vi "Read Constants.vi"(8 "error in (no error)":errorcluster, 11 "Tank Drive in":refnum<class "Tank Drive.lvclass">) -> (0 "error out":errorcluster, 2 "Constants":T1={"Drive Velocity Low Gear"={"P"=0.0, "I"=0.0, "D"=0.0, "F"=0.0, "integralZone"=0.0, "allowableClosedLoopError"=0, "maxIntegralAccumulator"=0.0, "closedLoopPeakOutput"=1.0, "closedLoopPeriod"=1}, "Drive Velocity High Gear"={"P"=0.0, "I"=0.0, "D"=0.0, "F"=0.0, "integralZone"=0.0, "allowableClosedLoopError"=0, "maxIntegralAccumulator"=0.0, "closedLoopPeakOutput"=1.0, "closedLoopPeriod"=1}, "Drive Motion Magic Primary Low Gear"={"P"=0.0, "I"=0.0, "D"=0.0, "F"=0.0, "integralZone"=0.0, "allowableClosedLoopError"=0, "maxIntegralAccumulator"=0.0, "closedLoopPeakOutput"=1.0, "closedLoopPeriod"=1}, "Drive Motion Magic Primary High Gear"={"P"=0.0, "I"=0.0, "D"=0.0, "F"=0.0, "integralZone"=0.0, "allowableClosedLoopError"=0, "maxIntegralAccumulator"=0.0, "closedLoopPeakOutput"=1.0, "closedLoopPeriod"=1}, "Drive Motion Magic Secondary Low Gear"={"P"=0.0, "I"=0.0, "D"=0.0, "F"=0.0, "integralZone"=0.0, "allowableClosedLoopError"=0, "maxIntegralAccumulator"=0.0, "closedLoopPeakOutput"=1.0, "closedLoopPeriod"=1}, "Drive Motion Magic Secondary High Gear"={"P"=0.0, "I"=0.0, "D"=0.0, "F"=0.0, "integralZone"=0.0, "allowableClosedLoopError"=0, "maxIntegralAccumulator"=0.0, "closedLoopPeakOutput"=1.0, "closedLoopPeriod"=1}, "Drive Sensors"={"Drive Right Invert"=FALSE, "Drive Right Sensor Phase"=FALSE, "Drive Left Invert"=FALSE, "Drive Left Sensor Phase"=FALSE}, "Motion Magic Constants"={"Low Gear Max Velocity"=0, "High Gear Max Velocity"=0, "Motion Magic Low Gear Max Velocity"=0, "Motion Magic Low Gear Max Acceleration"=0, "Motion Magic High Gear Max Velocity"=0, "Motion Magic High Gear Max Acceleration"=0}, "Supply Current Limit Configuration"={"Enable?"=FALSE, "Current Limit"=0.0, "Threshold Current"=0.0, "Threshold Time"=0.0}}, 3 "Tank Drive out":refnum<class "Tank Drive.lvclass">)   [LabVIEW 2019, in "Drive.lvlib" / "Tank Drive.lvclass"]
uses:
  Tank Drive.lvclass
  <vilib>/Rock Robotics/WPI/ThirdParty/Phoenix-LabVIEW/Motor Controller/Controls/CTRE_Phoenix_MotorControl_SlotStructure.ctl
  DriveOld/Controls/Drive Sensor Data.ctl
  DriveOld/Drive.lvclass
  DriveOld/Controls/Motion Magic Constants.ctl
  Controls/Constants.ctl
  <vilib>/Rock Robotics/WPI/ThirdParty/Phoenix-LabVIEW/Motor Controller/Controls/CTRE_Phoenix_MotorControl_SupplyCurrentLimitConfiguration.ctl
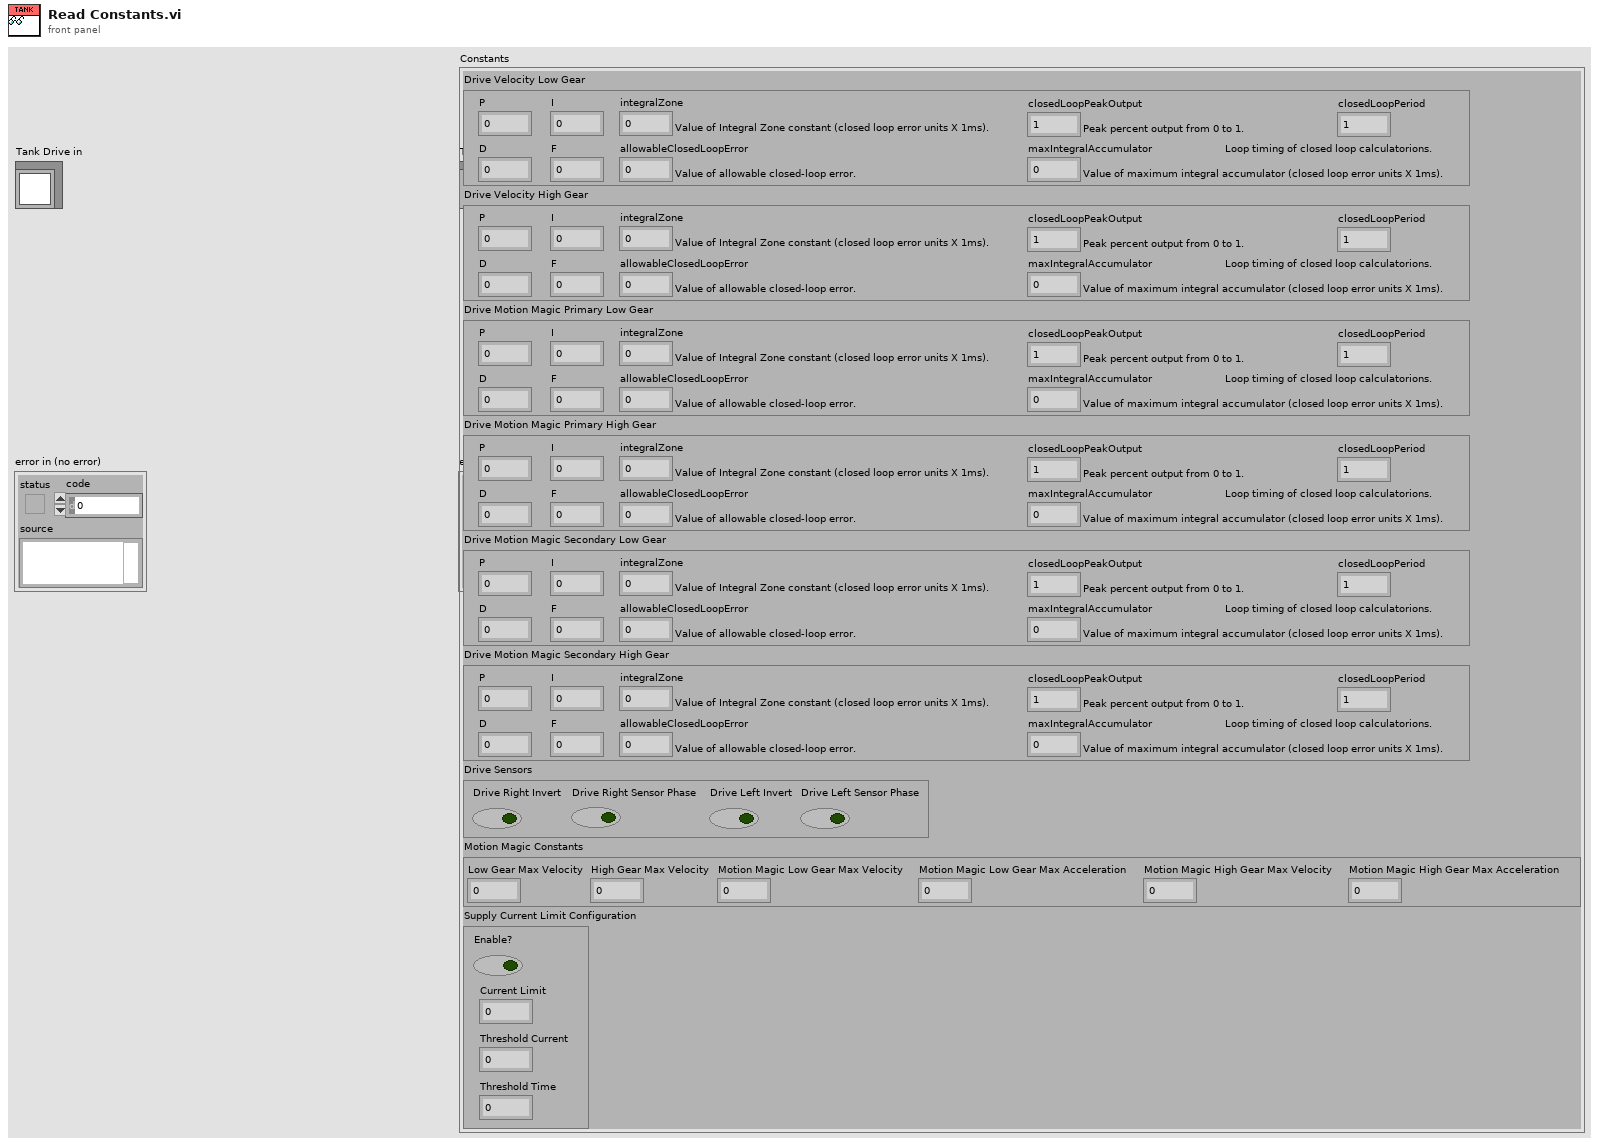
[diagram p1: front panel]
types:
  T1 = typedef "Drive.lvlib/Tank Drive.lvclass/Constants.ctl" = cluster{"Drive Velocity Low Gear":T2, "Drive Velocity High Gear":T2, "Drive Motion Magic Primary Low Gear":T2, "Drive Motion Magic Primary High Gear":T2, "Drive Motion Magic Secondary Low Gear":T2, "Drive Motion Magic Secondary High Gear":T2, "Drive Sensors":T3, "Motion Magic Constants":T4, "Supply Current Limit Configuration":T5}
  T2 = typedef "CTRE_Phoenix_MotorControl_SlotStructure.ctl" = cluster{"P":dbl, "I":dbl, "D":dbl, "F":dbl, "integralZone":dbl, "allowableClosedLoopError":i32, "maxIntegralAccumulator":dbl, "closedLoopPeakOutput":dbl, "closedLoopPeriod":i32}
  T3 = typedef "DriveOld.lvlib/Drive.lvclass/Drive Sensor Data.ctl" = cluster{"Drive Right Invert":bool, "Drive Right Sensor Phase":bool, "Drive Left Invert":bool, "Drive Left Sensor Phase":bool}
  T4 = typedef "DriveOld.lvlib/Drive.lvclass/Motion Magic Constants.ctl" = cluster{"Low Gear Max Velocity":u32, "High Gear Max Velocity":u32, "Motion Magic Low Gear Max Velocity":u32, "Motion Magic Low Gear Max Acceleration":u32, "Motion Magic High Gear Max Velocity":u32, "Motion Magic High Gear Max Acceleration":u32}
  T5 = typedef "CTRE_Phoenix_MotorControl_SupplyCurrentLimitConfiguration.ctl" = cluster{"Enable?":bool, "Current Limit":dbl, "Threshold Current":dbl, "Threshold Time":dbl}
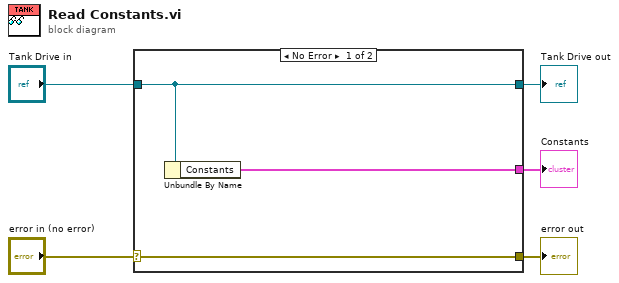
[diagram p0: block diagram]
diagram:
  n1 = case shown="No Error" "error in (no error)" {
    selector: "error in (no error)" -> [w8 w9]
    tunnel: [w8 w9] -> w4
    tunnel: [w7 w10] -> w2
    tunnel: "Tank Drive in" -> [w7 w10]
    tunnel: [w6 _] -> w1
    frame No Error {
      n2 = Unbundle By Name(w7) -> ("Constants"=w6:T1)
    }
    frame Error {
    }
  }
  "error out" <- w4
  "Tank Drive out" <- w2
  "Constants" <- w1
